vi "Is Dual Actuator.vi"(8 "error in (no error)":errorcluster, 11 "Model in":refnum<class "Model.lvclass">) -> (0 "error out":errorcluster, 2 "Is Dual Actuator":bool, 3 "Model out":refnum<class "Model.lvclass">)   [LabVIEW 2015, in "Model.lvclass"]
uses:
  Model.lvclass
  Typedefs/Actuator Types.ctl
  Model.lvclass/Model.ctl
  Typedefs/FAMT Typedefs.lvlib
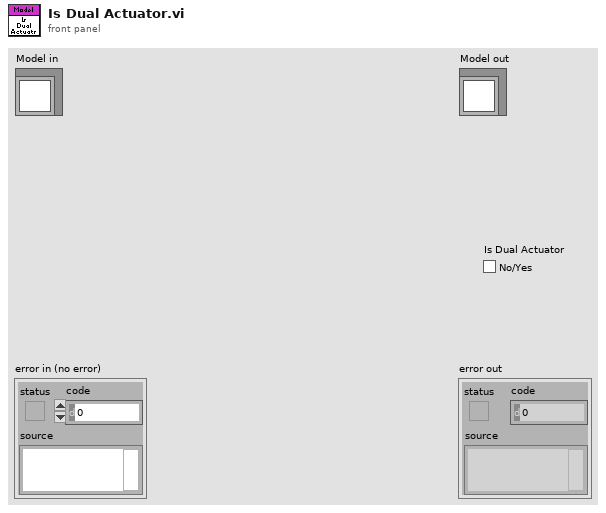
[diagram p1: front panel]
types:
  T1 = typedef "FAMT Typedefs.lvlib/Actuator Types.ctl" = enum16{"Single", "Dual", "Dual Outer"}
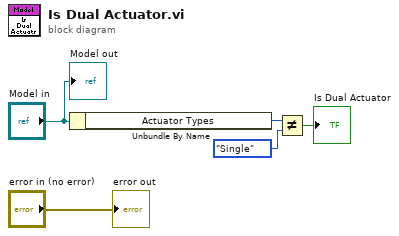
[diagram p0: block diagram]
diagram:
  n1 = Unbundle By Name("Model in") -> ("Actuator Types"=w3:T1)
  n2 = Not Equal?(x=w3, y=Actuator_Types."Single") -> (x != y?=→"Is Dual Actuator":bool)
  "error out" <- "error in (no error)"
  "Model out" <- "Model in"
